vi "Start Processs(static).vi"(8 "error in (no error)":errorcluster caption="错误输入（无错误）", 10 "fileName":string, 11 "ProcessClass 输入":refnum<class "ProcessClass.lvclass"> caption="DNL_LabVIEW Object in") -> (0 "error out":errorcluster caption="错误输出", 3 "ProcessClass 输出":refnum<class "ProcessClass.lvclass"> caption="DNL_LabVIEW Object out")   [LabVIEW 2012, in "ProcessClass.lvclass"]
uses:
  ProcessClass.lvclass
  ProcessClass.lvclass/ProcessClass.ctl
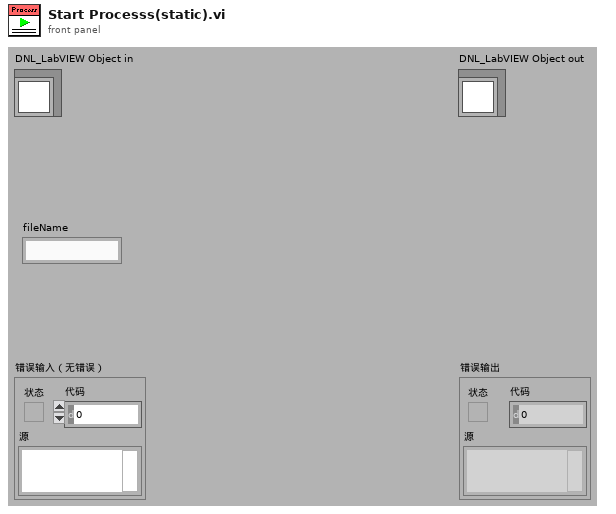
[diagram p1: front panel]
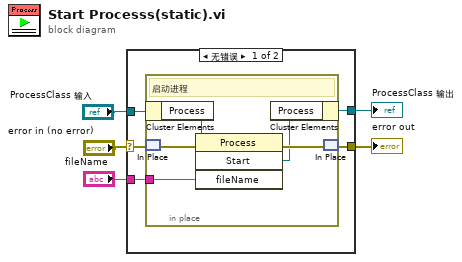
[diagram p0: block diagram]
diagram:
  n1 = case shown="无错误" "error in (no error)" {
    selector: "error in (no error)" -> [w10 w17]
    tunnel: [w9 w17] -> w4
    tunnel: [w6 w16] -> w2
    tunnel: "ProcessClass 输入" -> [w8 w16]
    tunnel: "fileName" -> [w7 _]
    frame No Error {
      n2 = in-place {
        in-place-border: w7 -> [w14]
        # "启动进程"
        n3 = in-place-cluster #1(w8) -> ("Process"=w15:refnum<k24>)
        n4 = in-place-match #2(w10) -> (w13:errorcluster)
        n5 = invoke class="Process" method="Start"(reference=w15, error in=w13, "fileName"=w14) -> (error out=w12:errorcluster, "Start"=w11:refnum<k24>)  [unwired: 1 in, 2 out]
        n6 = in-place-cluster #1("Process"=w11) -> (w6:refnum<class "ProcessClass.lvclass">)
        n7 = in-place-match #2(w12) -> (w9:errorcluster)
      }
    }
    frame Error {
    }
  }
  "error out" <- w4
  "ProcessClass 输出" <- w2
